vi "Set parameters.vi"(8 "error in (no error)":errorcluster caption="entrée d'erreur (pas d'erreur)", 11 "DelayLineLS4 en entrée":refnum<class "DLLS4.lvclass">) -> (0 "error out":errorcluster caption="sortie d'erreur", 3 "DelayLineLS4 en sortie":refnum<class "DLLS4.lvclass">)   [LabVIEW 2019, in "DLLS4.lvclass"]
uses:
  DLLS4.lvclass
  C:/Dev/TRANCON/Classes/Delay Line/DelayLine.lvclass
  C:/Dev/TRANCON/Classes/GeneralFunctionality/GeneralFunctionality.lvclass
  LS4 axis.ctl
  GeneralFunctionality/GeneralFunctionality.lvclass/GeneralFunctionality.ctl
  DelayLine.lvclass/DelayLine.ctl
  GeneralFunctionality/Read Config.vi
  Write wait ms.vi
  Config/Config.lvclass
  DelayLine.lvclass
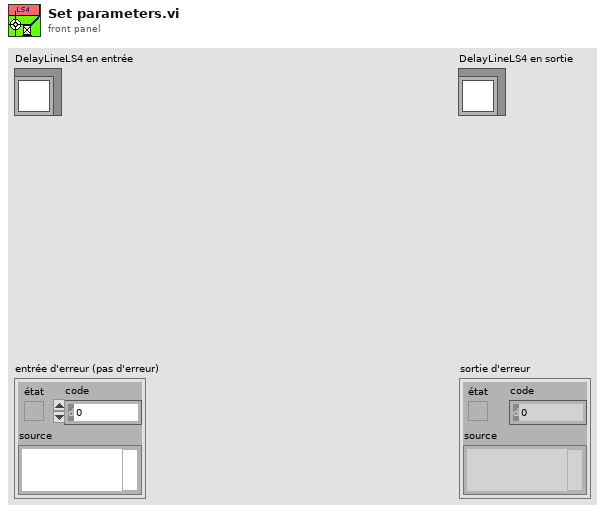
[diagram p1: front panel]
types:
  T1 = typedef "DelayLine.lvclass/LS4 axis.ctl" = u16
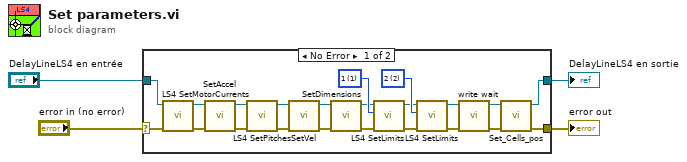
[diagram p0: block diagram]
diagram:
  n1 = case shown="No Error" "error in (no error)" {
    selector: "error in (no error)" -> [w21 w27]
    tunnel: [w7 w28] -> w4
    tunnel: "DelayLineLS4 en entrée" -> [w26 w28]
    tunnel: [w8 w27] -> w1
    frame No Error {
      w15 = T1 2 items=["1"=1, "2"=2, "3"=3, "4"=4] ("Axis")
      w16 = T1 1 items=["1"=1, "2"=2, "3"=3, "4"=4] ("Axis")
      n2 = call "LS4 SetMotorCurrents.vi"("error in (no error)"=w21, "DelayLineLS4 in"=w26) -> ("error out"=w20:errorcluster, "DelayLineLS4 out"=w25:refnum<class "DLLS4.lvclass">)  [unwired: 8 in]
      n3 = call "SetAccel.vi"("error in (no error)"=w20, "DelayLineLS4 in"=w25) -> ("error out"=w19:errorcluster, "DelayLineLS4 out"=w24:refnum<class "DLLS4.lvclass">)  [unwired: 8 in]
      n4 = call "LS4 SetPitches.vi"("error in (no error)"=w19, "DelayLineLS4 in"=w24) -> ("error out"=w18:errorcluster, "DelayLineLS4 out"=w23:refnum<class "DLLS4.lvclass">)  [unwired: 8 in]
      n5 = call "SetVel.vi"("error in (no error)"=w18, "DelayLineLS4 in"=w23) -> ("error out"=w17:errorcluster, "DelayLineLS4 out"=w22:refnum<class "DLLS4.lvclass">)  [unwired: 8 in]
      n6 = call "SetDimensions.vi"("error in (no error)"=w17, "DelayLineLS4 in"=w22) -> ("error out"=w11:errorcluster, "DelayLineLS4 out"=w14:refnum<class "DLLS4.lvclass">)  [unwired: 8 in]
      n7 = call "LS4 SetLimits.vi"("error in (no error)"=w11, "Axis"=w16, "DelayLineLS4 in"=w14) -> ("error out"=w12:errorcluster, "DelayLineLS4 out"=w13:refnum<class "DLLS4.lvclass">)  [unwired: 7 in]
      n8 = call "LS4 SetLimits.vi"("error in (no error)"=w12, "Axis"=w15, "DelayLineLS4 in"=w13) -> ("error out"=w9:errorcluster, "DelayLineLS4 out"=w10:refnum<class "DLLS4.lvclass">)  [unwired: 7 in]
      n9 = call "write wait.vi"("error in (no error)"=w9, "DelayLineLS4 en entrée"=w10) -> ("error out"=w6:errorcluster, "DelayLineLS4 en sortie"=w5:refnum<class "DLLS4.lvclass">)  [unwired: 8 in]
      n10 = call "Set_Cells_pos.vi"("error in (no error)"=w6, "DelayLine in"=w5) -> ("error out"=w8:errorcluster, "DelayLine out"=w7:refnum<class "DLLS4.lvclass">)  [unwired: 8 in]
    }
    frame Error {
    }
  }
  "error out" <- w1
  "DelayLineLS4 en sortie" <- w4
